vi "writeLJpinout.vi"() -> ()   [LabVIEW 2020]
uses:
  LJ Pin Setting.ctl
  <vilib>/addons/_JKI.lib/Serialization/JSON/JKI JSON Serialization.lvlib
panel:
  out "JSON String":string
  in  "LJ pinout":T1={"Ch1 Bias"="TDAC8", "Ch2 Bias"="TDAC9", "Ch3 Bias"="DAC0", "Ch4 Bias"="DAC1", "355 PWM"="DIO2", "AimingBeam PWM"="DIO3", "Laser Ready"="AIN0", "Interlock"="NOT USED", "Laser Start/Stop"="DIO15", "Red LED"="TDAC12", "Green LED"="TDAC13", "Foot Pedal"="DIO16"}
  # "Please use DIO names all the time. Using FIO or EIO will result in error. \nPlease use the pictures on right and bottom to decide what DIO number u are using.\nCopy and paste the following text to the setting file to change pin settings."
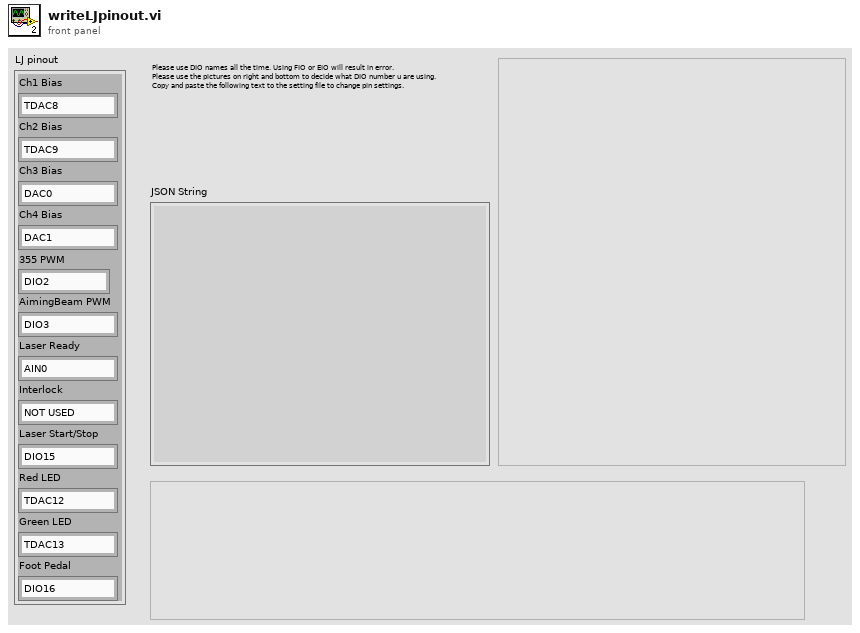
[diagram p1: front panel]
types:
  T1 = typedef "LJ Pin Setting.ctl" = cluster{"Ch1 Bias":string, "Ch2 Bias":string, "Ch3 Bias":string, "Ch4 Bias":string, "355 PWM":string, "AimingBeam PWM":string, "Laser Ready":string, "Interlock":string, "Laser Start/Stop":string, "Red LED":string, "Green LED":string, "Foot Pedal":string}
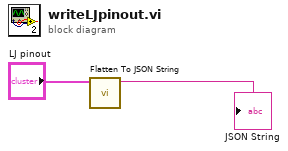
[diagram p0: block diagram]
diagram:
  n1 = call <vilib>:"Flatten To JSON String.vi"("Variant"="LJ pinout") -> ("JSON String"=→"JSON String":string)  [unwired: 9 in, 1 out]
